vi "GMonitor_Fengv2_Asylum.vi"(5 "Time Stamp":timestamp, 6 "v1":dbl[](array[numeric]) format="%#_6p", 7 "v0":dbl[](array[numeric]) format="%#_6p", 8 "lockin information":T1, 9 "tdms file":refnum<k34>) -> (0 "FtR":dbl, 1 "FtG":dbl, 2 "TtR":dbl, 3 "TtG":dbl, 4 "tdms file out":refnum<k34>)   [LabVIEW 2016]
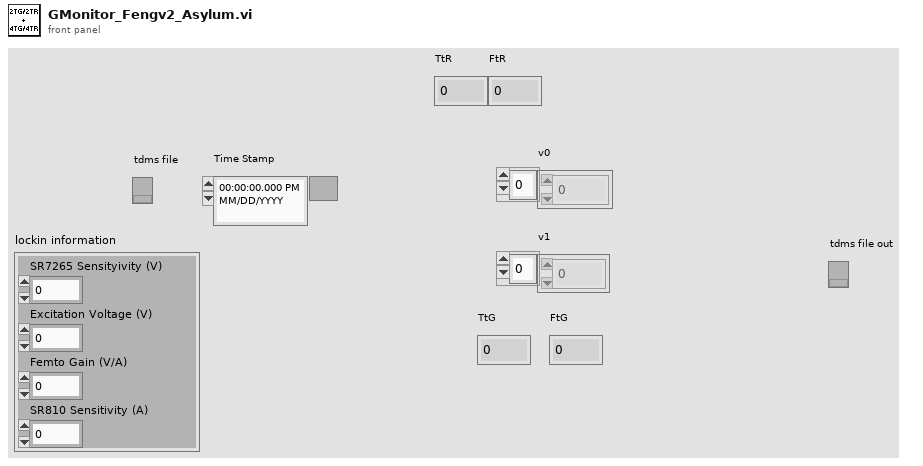
[diagram p1: front panel]
types:
  T1 = cluster{"SR7265 Sensityivity (V)":dbl, "Excitation Voltage (V)":dbl, "Femto Gain (V/A)":dbl, "SR810 Sensitivity (A)":dbl}
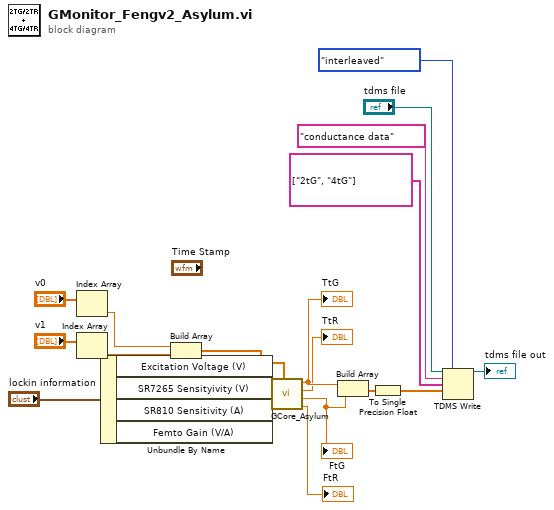
[diagram p0: block diagram]
diagram:
  n1 = Index Array(array="v0") -> (element=w6:dbl)  [unwired: 1 in]
  n2 = Index Array(array="v1") -> (element=w4:dbl)  [unwired: 1 in]
  n3 = Unbundle By Name("lockin information") -> ("Excitation Voltage (V)"=w12:dbl, "SR7265 Sensityivity (V)"=w11:dbl, "SR810 Sensitivity (A)"=w10:dbl, "Femto Gain (V/A)"=w9:dbl)
  n4 = Build Array(w6, w4) -> (w14:dbl[])
  n5 = call "GCore_Asylum.vi"("G data"=w14, "Femto Gain (V/A)"=w9, "SR830 sensitivity"=w10, "SR7265 sensitivity (V)"=w11, "Excitation voltage (V)"=w12) -> ("4tR"=→"FtR":dbl, "4tG"=w3:dbl, "2tR"=→"TtR":dbl, "2tG"=w8:dbl)
  "TtG" <- w8
  "FtG" <- w3
  n6 = Build Array(w8, w3) -> (w19:dbl[])
  n7 = To Single Precision Float(number=w19) -> (single precision float=w18:sgl[])
  n8 = TDMS Write(0:"tdms file", 1:enum16{"decimated", "interleaved"}."interleaved" ("data layout (0:decimated)"), 5:"conductance data", 7:string[] ["2tG", "4tG"], 9:w18) -> (4:→"tdms file out":refnum<k34>)  [unwired: 1 in, 3 out]
